vi "MSScript_Calc_GetParamArray.vi"(6 "Param":string[](array[string])) -> (0 "Is a variable?":bool[](array[boolean]), 1 "Value Error?":bool[](array[boolean]), 2 "Split Index":i32[](array[numeric]), 3 "ArrayVariable out":ext[](array[numeric]))   [LabVIEW 2018, in "MSScript.lvclass"]
uses:
  MSScript.lvclass
  MSScript_Transform_Extended.vi
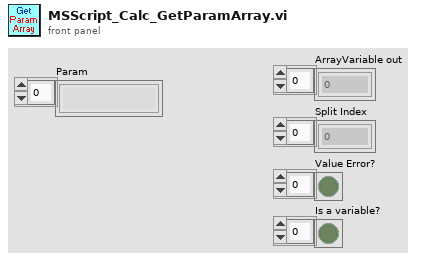
[diagram p1: front panel]
types:
  T1 = enum16{"Scalar", "ScalarArray", "Var", "VarArray", "Error"}
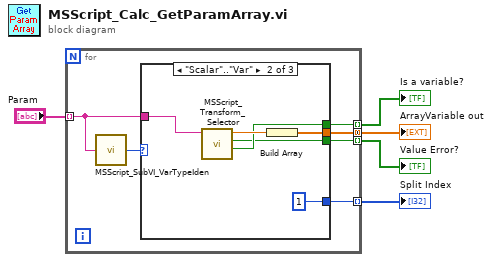
[diagram p0: block diagram]
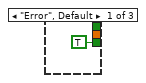
[diagram p2: hidden frame]
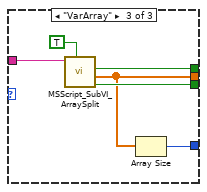
[diagram p3: hidden frame]
diagram:
  n1 = for {
    tunnel: "Param" -> [w7] mode=indexing
    tunnel: [w10] -> w3 mode=concatenating
    tunnel: [w9] -> w1 mode=indexing
    tunnel: [w8] -> w2 mode=indexing
    tunnel: [w6] -> w4 mode=indexing
    n2 = call "MSScript_SubVI_VarTypeIden.vi"("Var in"=w7) -> ("Type"=w11:T1)
    n3 = case shown="\"Scalar\"..\"Var\"" w11 {
      tunnel: [_ w17 w20] -> w10
      tunnel: [_ w16 w22] -> w9
      tunnel: [TRUE ("Value Error?") w15 w21] -> w8
      tunnel: w7 -> [_ w14 w23]
      tunnel: [_ 1 w19] -> w6
      frame "Error", Default {
      }
      frame "Scalar".."Var" {
        n4 = call-poly "MSScript_Transform_Selector.vi"("Check_Str"=w14) -> ("Is a variable ?"=w16:bool, "Value Error?"=w15:bool, "Value Output"=w18:ext)  [unwired: 8 in]
        n5 = Build Array(w18) -> (w17:ext[])
      }
      frame "VarArray" {
        n6 = call "MSScript_SubVI_ArraySplit.vi"("GetValue? (F)"=TRUE, "VarString in"=w23) -> ("Value Error?"=w21:bool, "ArrayVariable out"=w20:ext[], "Is a variable?"=w22:bool)  [unwired: 6 in, 1 out]
        n7 = Array Size(array=w20) -> (size(s)=w19:i32)
      }
    }
  }
  "Value Error?" <- w2
  "Is a variable?" <- w1
  "ArrayVariable out" <- w3
  "Split Index" <- w4
